vi "10.-Format Into String.vi"() -> ()   [LabVIEW 2020]
panel:
  out "length":i32
  out "concatenated string":string
  in  "Unidad":string
  in  "Encabezado":string
  in  "Numero":dbl format="%#_13g"
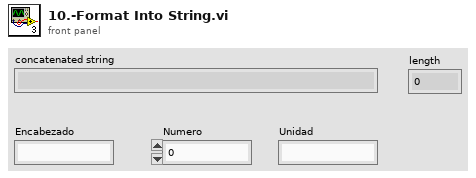
[diagram p1: front panel]
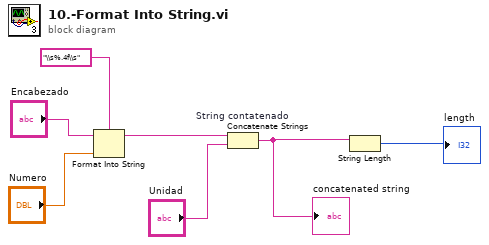
[diagram p0: block diagram]
diagram:
  n1 = Format Into String "Format Into String"(format string="\\s%.4f\\s", initial string="Encabezado", "Numero") -> (resulting string=w4:string)  [unwired: 1 in, 1 out]
  n2 = Concatenate Strings "String contatenado"(w4, "Unidad") -> (w2:string)
  "concatenated string" <- w2
  n3 = String Length(string=w2) -> (length=→"length":i32)
